vi "Save-available-maps.vi"(8 "error in":errorcluster, 11 "Data ref. in":refnum<data-value>) -> (0 "error IO":errorcluster, 3 "Data ref.":refnum<data-value>)   [LabVIEW 2013, in "CameraVision.lvlib" / "CV-Storage.lvclass"]
uses:
  CV-Storage.lvclass
  CV-Main.lvclass
  CV-Main.lvclass/CV-Main.ctl
  Mapping/CV-Mapping.lvclass/CV-Mapping.ctl
  CV-Storage.lvclass/CV-Storage.ctl
  UI/Camera-selector.ctl
  Read Characteristics file reference RW.vi
  Read Storage labels.vi
  Read Save what.vi
  Mapping/Read Available.vi
  Read Storage params.vi
  Read Mapping params.vi
  Mapping/CV-Mapping.lvclass
  UI/CV-UI.lvclass
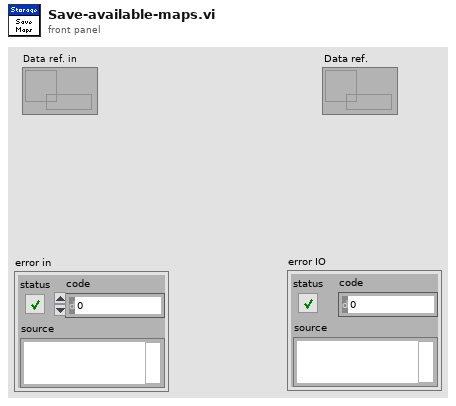
[diagram p1: front panel]
types:
  T1 = typedef "CameraVision.lvlib/CV-UI.lvclass/Camera-selector.ctl" = enum16{"Camera 1", "Camera 2"}
  T2 = typedef "CameraVision.lvlib/Mapping.lvclass/Mapping-characteristic.ctl" = enum16{"Average intensity [0-255]", "Peak intensity [0-255]", "Melt-pool size [mm²]", "Melt-pool aspect ratio []", "Melt-pool fragments []", "Average temperature [°C]", "Max. temperature [°C]", "Min. temperature [°C]", "Std. dev. temperature [°C]"}
  T3 = typedef "CameraVision.lvlib/Storage.lvclass/Storage-types-labels.ctl" = cluster{"Original":string, "Corrected":string, "Binary":string, "Temperature":string, "Characteristics":string, "Mapping":string, "TemperatureValues":string}
  T4 = cluster{"Original":bool, "Corrected":bool, "Binary":bool, "Temperature":bool, "Characteristics":bool, "Mapping":bool, "TemperatureValues":bool}
  T5 = cluster{"Signal":sgl[], "Xcoords":sgl[], "Ycoords":sgl[]}
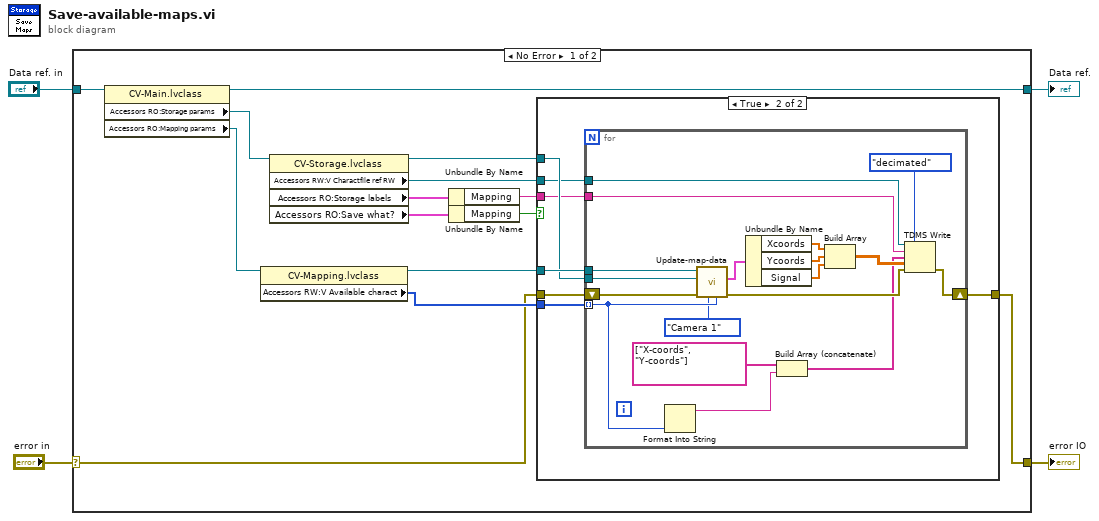
[diagram p0: block diagram]
diagram:
  n1 = case shown="No Error" "error in" {
    selector: "error in" -> [w9 w46]
    tunnel: [w18 w46] -> w4
    tunnel: "Data ref. in" -> [w8 w45]
    tunnel: [w5 w45] -> w1
    frame No Error {
      n2 = property class="CV-Main.lvclass"(reference=w8) -> (reference out=w5:refnum<data-value>, "Accessors RO:Storage params"=w6:refnum<data-value>, "Accessors RO:Mapping params"=w7:refnum<data-value>)  [unwired: 1 in, 1 out]
      n3 = property class="CV-Mapping.lvclass"(reference=w7) -> (reference out=w11:refnum<data-value>, "Accessors RW:V Available charact"=w10:T2[])  [unwired: 1 in, 1 out]
      n4 = property class="CV-Storage.lvclass"(reference=w6) -> (reference out=w12:refnum<data-value>, "Accessors RW:V Charactfile ref RW"=w17:refnum<k34>, "Accessors RO:Storage labels"=w16:T3, "Accessors RO:Save what?"=w14:T4)  [unwired: 1 in, 1 out]
      n5 = Unbundle By Name(w16) -> ("Mapping"=w15:string)
      n6 = Unbundle By Name(w14) -> ("Mapping"=w13:bool)
      n7 = case shown="True" w13 {
        tunnel: [w19 w21] -> w18
        tunnel: w9 -> [w19 w24]
        tunnel: w17 -> [_ w23]
        tunnel: w15 -> [_ w22]
        tunnel: w11 -> [_ w26]
        tunnel: w12 -> [_ w25]
        tunnel: w10 -> [_ w20]
        frame False {
        }
        frame True {
          n8 = for {
            tunnel: w26 -> [w44]
            tunnel: w25 -> [w43]
            tunnel: w23 -> [w41]
            tunnel: w22 -> [w40]
            tunnel: w20 -> [w28] mode=indexing
            shift-right: [w33] -> w21
            shift-left: w24 -> [w42]
            n9 = Format Into String(w28) -> (resulting string=w30:string)  [unwired: 3 in, 1 out]
            n10 = call "Update-map-data.vi"("Active characteristic"=w28, "Active camera"=Camera-selector."Camera 1", "error in"=w42, "Storage params. ref."=w43, "Mapping params. ref. in"=w44) -> ("error IO"=w39:errorcluster, "Map"=w37:T5)  [unwired: 4 in, 1 out]
            n11 = Unbundle By Name(w37) -> ("Xcoords"=w35:sgl[], "Ycoords"=w36:sgl[], "Signal"=w32:sgl[])
            n12 = Build Array (concatenate)(string[] ["X-coords", "Y-coords"] ("channel name(s) in (Untitled)"), w30) -> (w29:string[])
            n13 = Build Array(w35, w36, w32) -> (w34:sgl[][])
            n14 = TDMS Write(0:w41, 1:enum16{"decimated", "interleaved"}."decimated" ("data layout (0:decimated)"), 5:w40, 7:w29, 9:w34, 11:w39) -> (15:w33:errorcluster)  [unwired: 3 out]
          }
        }
      }
    }
    frame Error {
    }
  }
  "error IO" <- w4
  "Data ref." <- w1
